vi "get Number Of SADI.vi"() -> (3 "function return":u32)   [LabVIEW 2025, in "SADI_FW3.lvlib"]
doc: "SADI_API unsigned int getNumberOfSADI();"
uses:
  SADI_FW3.lvlib
  SADI_FW3.dll
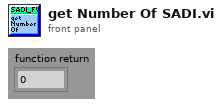
[diagram p1: front panel]
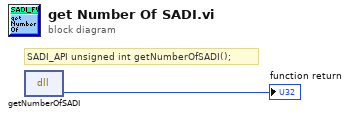
[diagram p0: block diagram]
diagram:
  # "SADI_API unsigned int getNumberOfSADI();"
  n1 = dll-call lib="C:/Users/noaht/School/Fall 2025/Controls Lab/Lab 3/EML4314c_FA25_framework_0/LVLib/SADI_FW3.*" fn="getNumberOfSADI"() -> (→"function return":u32)  [unwired: 3 in, 2 out]
